vi "windows_heater.vi"(1 "Stop! Refnum":refnum<vi>, 2 "Switch Refnum":refnum<vi>, 3 "Window Heater Switch":tag) -> ()   [LabVIEW 2017]
uses:
  <vilib>/DAQmx/write.llb/DAQmx Write (Analog DBL 1Chan 1Samp).vi
  <vilib>/DAQmx/create/channels.llb/DAQmx Create Channel (AO-Voltage-Basic).vi
  <vilib>/DAQmx/miscellaneous.llb/DAQmx Fill In Error Info.vi
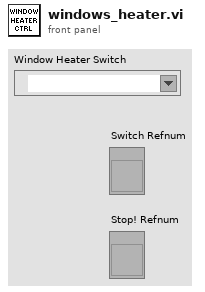
[diagram p1: front panel]
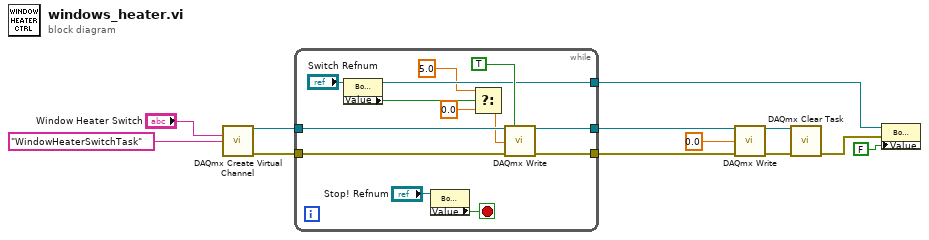
[diagram p0: block diagram]
diagram:
  n1 = call-poly <vilib>:"DAQmx Create Virtual Channel.vi"("physical channels"="Window Heater Switch", "name to assign"="WindowHeaterSwitchTask") -> ("task out"=w12:refnum<k21>, "error out"=w11:errorcluster)  [unwired: 12 in]
  n2 = while {
    tunnel: w12 -> [w23]
    tunnel: w11 -> [w22]
    tunnel: [w19] -> w3
    tunnel: [w18] -> w2
    tunnel: [w17] -> w8
    stop <- w24 stop-if-true
    n3 = property class="Bool (strict)"(reference="Switch Refnum") -> (reference out=w17:refnum<vi>, "Value"=w16:bool)  [unwired: 1 in, 1 out]
    n4 = property class="Bool (strict)"(reference="Stop! Refnum") -> ("Value"=w24:bool)  [unwired: 1 in, 2 out]
    n5 = Select(t=5.0, s=w16, f=0.0) -> (s? t:f=w13:dbl)
    n6 = call-poly <vilib>:"DAQmx Write.vi"("task/channels in"=w23, "auto start"=TRUE, "data"=w13, "error in"=w22) -> ("task out"=w19:refnum<k21>, "error out"=w18:errorcluster)  [unwired: 9 in, 1 out]
  }
  n7 = call-poly <vilib>:"DAQmx Write.vi"("task/channels in"=w3, "data"=0.0, "error in"=w2) -> ("task out"=w5:refnum<k21>, "error out"=w4:errorcluster)  [unwired: 10 in, 1 out]
  n8 = call <vilib>:"DAQmx Clear Task.vi"("task in"=w5, "error in"=w4) -> ("error out"=w7:errorcluster)  [unwired: 13 in]
  n9 = property class="Bool (strict)"(reference=w8, error in=w7, "Value"=FALSE) -> ()  [unwired: 2 out]
